vi "Convert Data to TDMS format.vi"(10 "Data":dbl[](array[numeric]), 11 "Mode":string) -> (2 "Data Out":dbl[][](array[numeric]) format="%#.3g", 3 "Array out":string[][](array[string]))   [LabVIEW 2020, in "SAVE.lvlib"]
uses:
  SAVE.lvlib
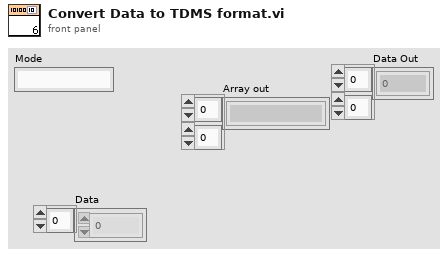
[diagram p1: front panel]
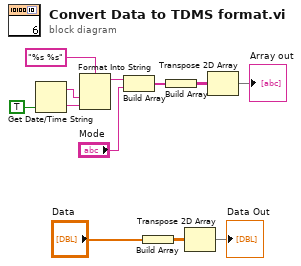
[diagram p0: block diagram]
diagram:
  n1 = Get Date/Time String(want seconds? (F)=TRUE) -> (date string=w8:string, time string=w9:string)  [unwired: 2 in]
  n2 = Format Into String(format string="%s %s", w8, w9) -> (resulting string=w5:string)  [unwired: 2 in, 1 out]
  n3 = Build Array(w5, "Mode") -> (w11:string[])
  n4 = Build Array("Data") -> (w2:dbl[][])
  n5 = Build Array(w11) -> (w10:string[][])
  n6 = Transpose 2D Array(2D array=w2) -> (transposed array=→"Data Out":dbl[][])
  n7 = Transpose 2D Array(2D array=w10) -> (transposed array=→"Array out":string[][])
